vi "ZC_didian.vi"(0 "action":string, 1 "LabVIEW Web Service Request":refnum<class "Web Request.lvclass"> caption="LabVIEW Web服务请求", 2 "zrren":string, 3 "beizhu":string, 5 "id":string, 7 "name":string, 9 "number":string, 11 "weizhi":string, 14 "key":string) -> (6 "error":errorcluster)   [LabVIEW 2017]
uses:
  <vilib>/wsapi/Web Request.lvclass
panel:
  out "postdata":string caption="post数据"
  out "error out":errorcluster caption="错误输出"
  # "Web服务请求输入接线端用于调用“Web服务”选板的VI。除非不需要访问该选板，否则不要在连线板上删除这个输入接线端。"
  # "添加至连线板的每一个其他输入控件，在URL中对应于一个输入。如需在接线端模式输出（默认设置）下包含显示控件，则该显示控件必须与连线板相连。"
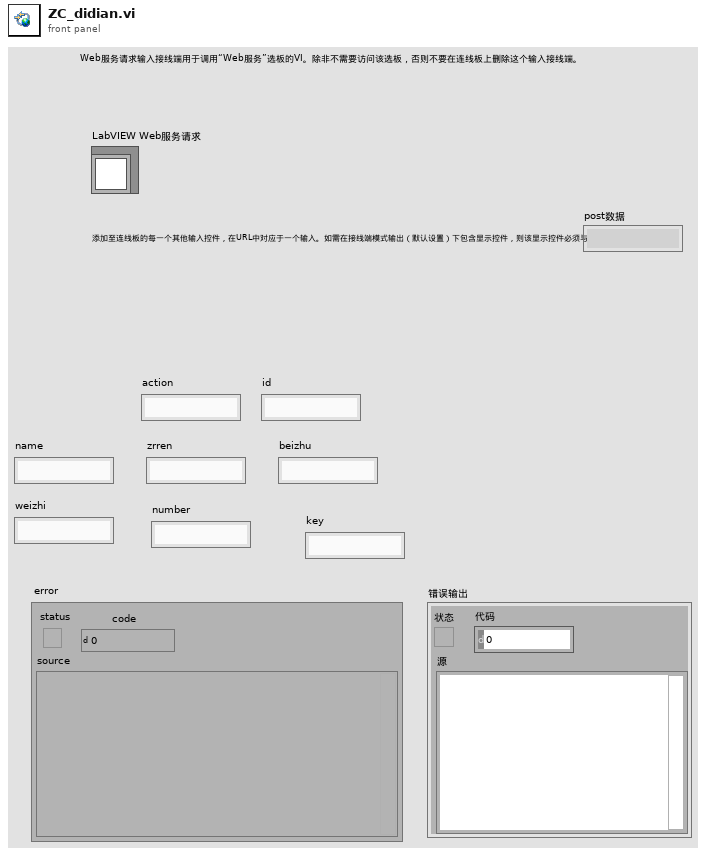
[diagram p1: front panel]
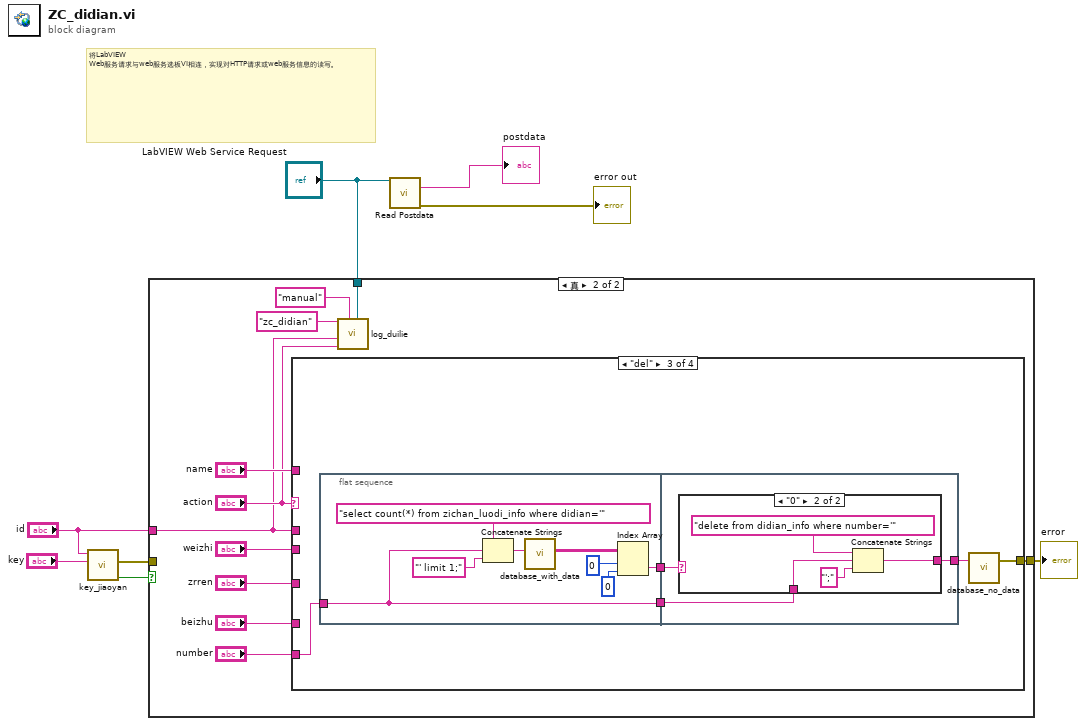
[diagram p0: block diagram]
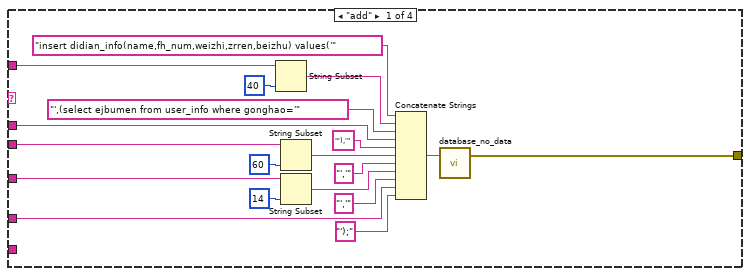
[diagram p3: hidden frame]
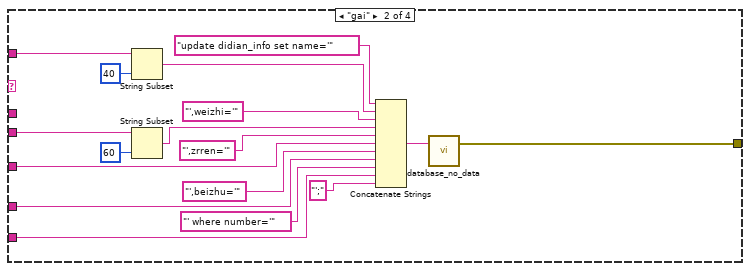
[diagram p4: hidden frame]
diagram:
  # "将LabVIEW Web服务请求与web服务选板VI相连，实现对HTTP请求或web服务信息的读写。"
  n1 = call "key_jiaoyan.vi"("key_client"="key", "gonghao"="id") -> ("jy"=w2:bool, "error"=w1:errorcluster)  [unwired: 8 in]
  n2 = case shown="真" w2 {
    tunnel: [w9 w20] -> w7
    tunnel: "LabVIEW Web Service Request" -> [_ w12]
    tunnel: "id" -> [_ w10]
    tunnel: w1 -> [w9 _]
    frame False {
    }
    frame True {
      n3 = case shown="\"del\"" "action" {
        tunnel: [w27 w56 w61 _] -> w20
        tunnel: "beizhu" -> [w26 w43 _ _]
        tunnel: "zrren" -> [w25 w44 _ _]
        tunnel: "weizhi" -> [w24 w45 _ _]
        tunnel: "name" -> [w23 w46 _ _]
        tunnel: w10 -> [w21 _ _ _]
        tunnel: "number" -> [_ w41 w58 _]
        frame "add" {
          n4 = String Subset(string=w23, length (rest)=40 ("长度（剩余）")) -> (substring=w36:string)  [unwired: 1 in]
          n5 = String Subset(string=w24, length (rest)=60 ("长度（剩余）")) -> (substring=w34:string)  [unwired: 1 in]
          n6 = String Subset(string=w25, length (rest)=14 ("长度（剩余）")) -> (substring=w30:string)  [unwired: 1 in]
          n7 = Concatenate Strings("insert didian_info(name,fh_num,weizhi,zrren,beizhu) values('" ("格式字符串"), w36, "',(select ejbumen from user_info where gonghao='" ("字符串"), w21, "'),'" ("字符串"), w34, "','" ("字符串"), w30, "','" ("字符串"), w26, "');" ("字符串")) -> (w28:string)
          n8 = call "database_no_data.vi"("input"=w28) -> ("error"=w27:errorcluster)  [unwired: 2 in]
        }
        frame "gai" {
          n9 = String Subset(string=w46, length (rest)=40 ("长度（剩余）")) -> (substring=w54:string)  [unwired: 1 in]
          n10 = String Subset(string=w45, length (rest)=60 ("长度（剩余）")) -> (substring=w55:string)  [unwired: 1 in]
          n11 = Concatenate Strings("update didian_info set name='" ("格式字符串"), w54, "',weizhi='" ("字符串"), w55, "',zrren='" ("字符串"), w44, "',beizhu='" ("字符串"), w43, "' where number='" ("字符串"), w41, "';" ("字符串")) -> (w47:string)
          n12 = call "database_no_data.vi"("input"=w47) -> ("error"=w56:errorcluster)  [unwired: 2 in]
        }
        frame "del" {
          n13 = flat-sequence {
            tunnel: w58 -> [w67]
            tunnel: [w67] -> w60
            tunnel: [w62] -> w59
            tunnel: [w72] -> w57
            tunnel: w60 -> [w71]
            tunnel: w59 -> [w70]
            frame #0 {
              n14 = Concatenate Strings("select count(*) from zichan_luodi_info where didian='" ("格式字符串"), w67, "' limit 1;" ("字符串")) -> (w66:string)
              n15 = call "database_with_data.vi"("input"=w66) -> ("Data"=w63:string[][])  [unwired: 9 in, 1 out]
              n16 = Index Array(array=w63, index (row)=0 ("索引 (行)"), index (col)=0 ("禁用的索引 (列)")) -> (element=w62:string)
            }
            frame #1 {
              n17 = case shown="\"0\"" w70 {
                tunnel: [_ w74] -> w72
                tunnel: w71 -> [_ w73]
                frame "假", Default {
                }
                frame "0" {
                  n18 = Concatenate Strings("delete from didian_info where number='" ("格式字符串"), w73, "';" ("字符串")) -> (w74:string)
                }
              }
            }
          }
          n19 = call "database_no_data.vi"("input"=w57) -> ("error"=w61:errorcluster)  [unwired: 2 in]
        }
        frame Default {
        }
      }
      n20 = call "log_duilie.vi"("LabVIEW Web Service Request"=w12, "type"="manual", "action"="action", "user"=w10, "yw"="zc_didian") -> ()  [unwired: 7 in]
    }
  }
  "error" <- w7
  n21 = call <vilib>:"Read Postdata.vi"("LabVIEW Web Service Request"="LabVIEW Web Service Request") -> ("postdata"=→"postdata":string, "error out"=→"error out":errorcluster)  [unwired: 12 in, 1 out]
